vi "总磷总氮启动参数对话框.vi"() -> (2 "确认":bool, 3 "元素":cluster{"命令":string, "data":variant})   [LabVIEW 2016, in "斯坦道总磷总氮.lvlib"]
panel:
  out "标液值":dbl caption="标液值："
  in  "取消":bool
  in  "确定":bool
  in  "测量间隔":u16
  in  "模式设置":T1(ring)
  in  "量程切换":u16(ring)=2 items=["H", "L", "AUTO"]
  in  "站号":u16(ring)=1 items=["总磷"=1, "总氮"=2]
  in  "控制命令":T2(ring)
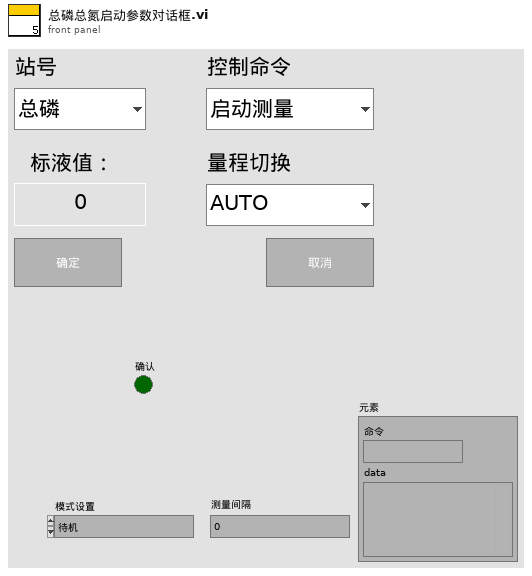
[diagram p1: front panel]
types:
  T1 = enum16{"待机", "连续模式", "周期模式", "定点模式", "受控模式", "手动模式"}
  T2 = enum16{"启动测量", "标样核查", "零点核查", "跨度核查", "空白测试", "平行样测试", "加标回收", "空白校准", "标样校准", "初始化（清洗）", "停止测试", "仪器重启", "校时", "模式设置", "测量间隔设置"}
  T3 = cluster{"站号":u16, "量程切换":enum32{"H", "L", "AUTO"}, "控制命令":enum16{"启动测量", "标样核查", "零点核查", "跨度核查", "空白测试", "平行样测试", "加标回收", "空白校准", "标样校准", "初始化（清洗）", "停止测试", "仪器重启", "校时", "模式设置", "测量间隔设置", "盲样测试"}, "模式设置":enum16{"待机", "连续模式", "周期模式", "定点模式", "受控模式", "手动模式"}, "测量间隔":u16}
  T4 = cluster{"总磷跨度值":dbl, "总磷零点标准液浓度":dbl, "总磷跨度标准液浓度":dbl, "总磷标准液标准浓度":dbl, "总氮跨度值":dbl, "总氮零点标准液浓度":dbl, "总氮跨度标准液浓度":dbl, "总氮标准液标准浓度":dbl}
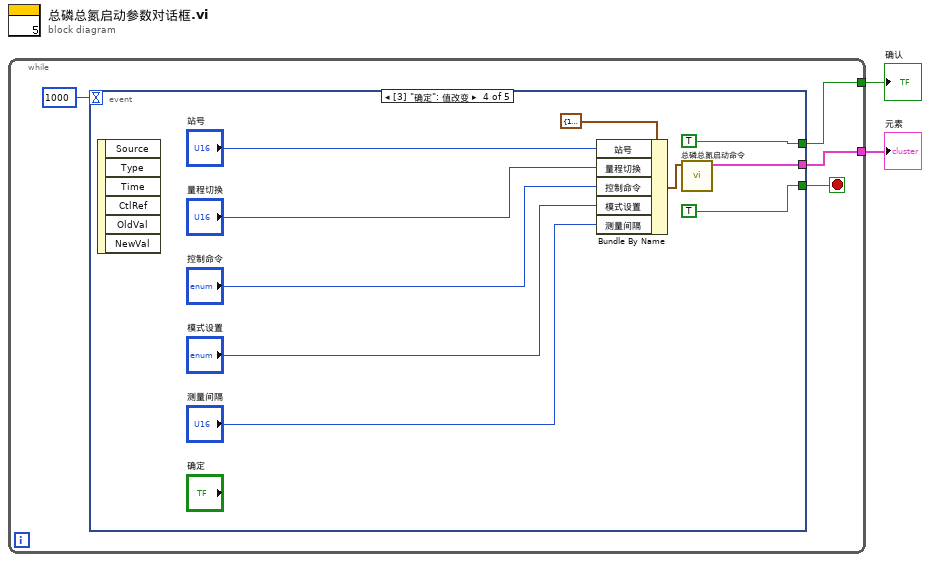
[diagram p0: block diagram]
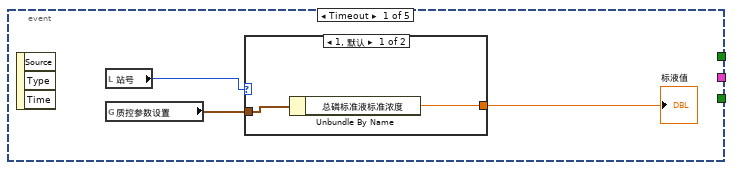
[diagram p2: hidden frame]
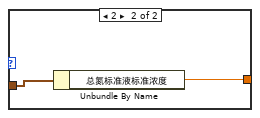
[diagram p3: hidden frame]
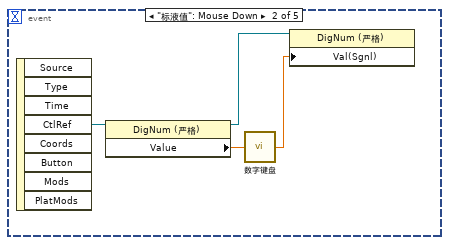
[diagram p4: hidden frame]
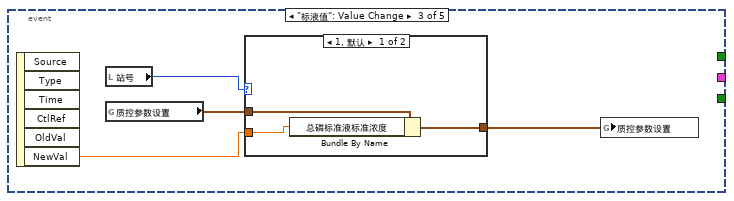
[diagram p5: hidden frame]
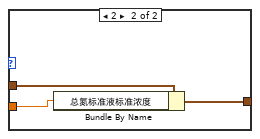
[diagram p6: hidden frame]
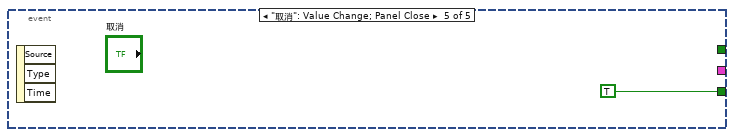
[diagram p7: hidden frame]
diagram:
  n1 = while {
    tunnel: [w4] -> w2
    tunnel: [w3] -> w1
    stop <- w6 stop-if-true
    n2 = event shown="[3] \"确定\": 值改变" {
      selector: _ -> [_ _ _ _ _]
      dyn-events: _ -> [_ _ _ _ _]
      timeout: 1000 -> [_ _ _ _ _]
      tunnel: [_ _ _ TRUE TRUE] -> w6
      tunnel: [_ _ _ TRUE _] -> w4
      tunnel: [_ _ _ w35 _] -> w3
      event Timeout {
        n3 = event-data() -> ()  [unwired: 1 in, 3 out]
        n4 = local read "站号"() -> (w8:u16)
        n5 = global read "总磷总氮断电保存全局变量.vi" "质控参数设置"() -> (w9:T4)
        n6 = case shown="1, 默认" w8 {
          tunnel: w9 -> [w11 w13]
          tunnel: [w10 w12] -> w7
          frame 1, Default {
            n7 = Unbundle By Name(w11) -> ("总磷标准液标准浓度"=w10:dbl)
          }
          frame 2 {
            n8 = Unbundle By Name(w13) -> ("总氮标准液标准浓度"=w12:dbl)
          }
        }
        "标液值" <- w7
      }
      event "标液值": Mouse Down {
        n9 = event-data() -> ("CtlRef"=w17:refnum<vi>)  [unwired: 1 in, 7 out]
        n10 = property class="DigNum (严格)"(reference=w17) -> (reference out=w14:refnum<vi>, "Value"=w16:dbl)  [unwired: 1 in, 1 out]
        n11 = call "数字键盘.vi"("OldNumber"=w16) -> ("NewNumber"=w15:dbl)
        n12 = property class="DigNum (严格)"(reference=w14, "Val(Sgnl)"=w15) -> ()  [unwired: 1 in, 2 out]
      }
      event "标液值": Value Change {
        n13 = event-data() -> ("NewVal"=w19:dbl)  [unwired: 1 in, 5 out]
        n14 = local read "站号"() -> (w21:u16)
        n15 = global read "总磷总氮断电保存全局变量.vi" "质控参数设置"() -> (w20:T4)
        n16 = case shown="1, 默认" w21 {
          tunnel: w20 -> [w24 w27]
          tunnel: [w22 w25] -> w18
          tunnel: w19 -> [w23 w26]
          frame 1, Default {
            n17 = Bundle By Name(cluster=w24, "总磷标准液标准浓度"=w23) -> (w22:T4)
          }
          frame 2 {
            n18 = Bundle By Name(cluster=w27, "总氮标准液标准浓度"=w26) -> (w25:T4)
          }
        }
        n19 = global write "总磷总氮断电保存全局变量.vi" "质控参数设置"(w18) -> ()
      }
      event "确定": Value Change {
        n20 = event-data() -> ()  [unwired: 1 in, 6 out]
        n21 = Bundle By Name(cluster=T3 {"站号"=1, "量程切换"=enum."AUTO", "控制命令"=enum."启动测量", "模式设置"=enum."待机", "测量间隔"=0} ("参数"), "站号"="站号", "量程切换"="量程切换", "控制命令"="控制命令", "模式设置"="模式设置", "测量间隔"="测量间隔") -> (w33:T3)
        n22 = call "总磷总氮启动命令.vi"("参数"=w33) -> ("启动命令"=w35:cluster{"命令":string, "data":variant})  [unwired: 10 in]
      }
      event "取消": Value Change; Panel Close {
        n23 = event-data() -> ()  [unwired: 1 in, 3 out]
      }
    }
  }
  "元素" <- w1
  "确认" <- w2
